vi "Draw Realtime.vi"(4 "Queue Items":i32, 5 "ColorRamp in":refnum<vi>, 6 "3D":T2, 7 "Resolution":i32=444, 8 "error in (no error)":errorcluster, 9 "Litho Point Old":T3, 10 "Litho Point":T3, 11 "Image in":T1(plugin-control)) -> (0 "error out":errorcluster, 3 "Image out":T1)   [LabVIEW 2016]
doc: "This VI draws on the realtime 2D and 3D images."
uses:
  <vilib>/vision/Image Controls.llb/IMAQ Image.ctl
  <vilib>/picture/3D Picture Control/Helpers/Apply Texture (no reference).vi
  <vilib>/picture/3D Picture Control/NI_3D Picture Control.lvlib
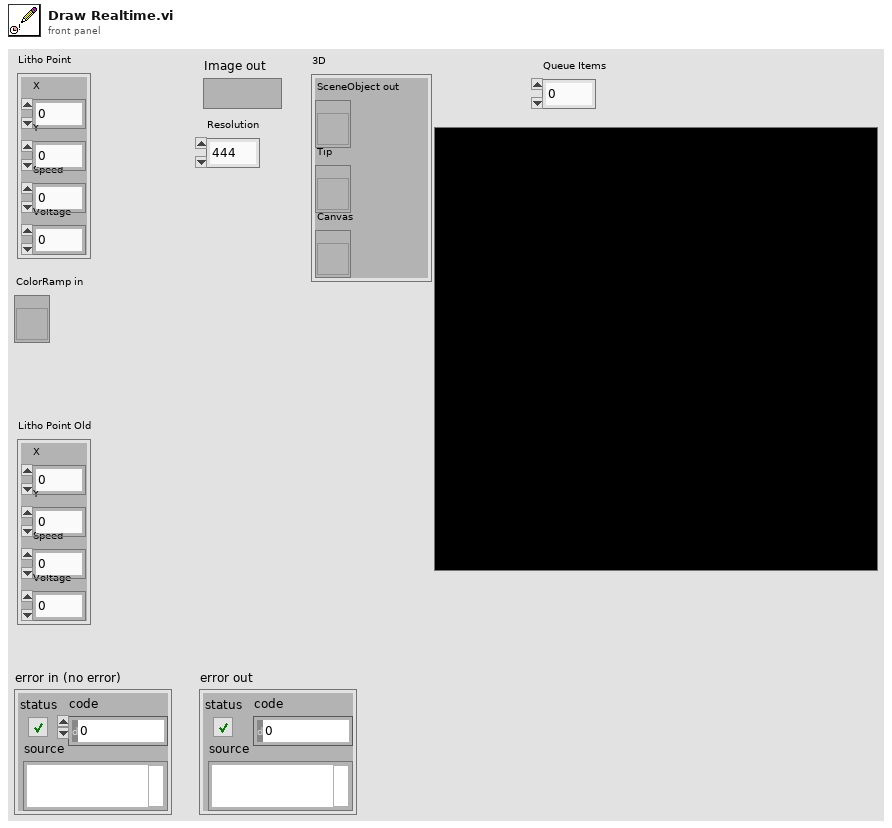
[diagram p1: front panel]
types:
  T1 = typedef "IMAQ Image.ctl" = refnum<image>
  T2 = cluster{"SceneObject out":refnum<vi>, "Tip":refnum<vi>, "Canvas":refnum<vi>}
  T3 = cluster{"X":dbl, "Y":dbl, "Speed":dbl, "Voltage":dbl}
  T4 = typedef "imagedata.ctl" = cluster{"image type":i32, "image depth":i32, "image":u8[], "mask":u8[], "colors":u32[], "Rectangle":cluster{"left":i16, "top":i16, "right":i16, "bottom":i16}}
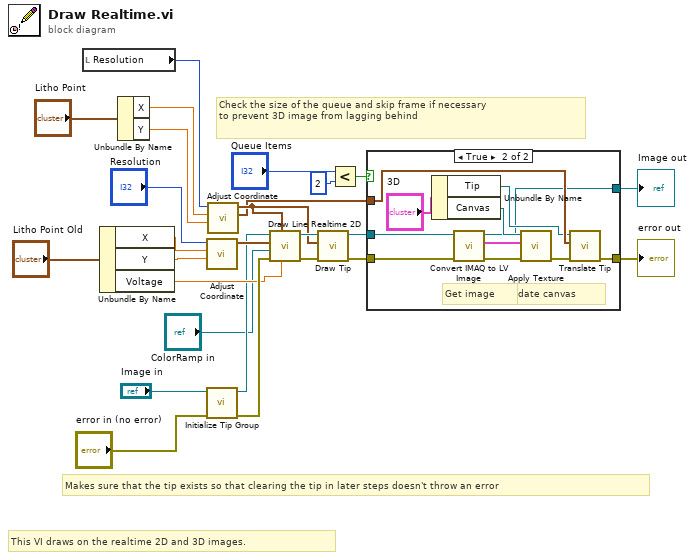
[diagram p0: block diagram]
diagram:
  # "This VI draws on the realtime 2D and 3D images."
  # "Makes sure that the tip exists so that clearing the tip in later steps doesn't throw an error"
  # "Check the size of the queue and skip frame if necessary\nto prevent 3D image from lagging behind"
  n1 = local read "Resolution"() -> (w3:i32)
  n2 = Unbundle By Name("Litho Point Old") -> ("X"=w24:dbl, "Y"=w25:dbl, "Voltage"=w12:dbl)
  n3 = Unbundle By Name("Litho Point") -> ("X"=w10:dbl, "Y"=w9:dbl)
  n4 = call "Adjust Coordinate.vi"("Y"=w25, "X"=w24, "Resolution"="Resolution") -> ("Adjusted Coordinate"=w23:cluster{dbl, dbl})  [unwired: 7 in, 1 out]
  n5 = call "Initialize Tip Group.vi"("error in (no error)"="error in (no error)", "Refnum in"="Image in") -> ("error out"=w19:errorcluster, "Refnum out"=w5:T1)  [unwired: 8 in]
  n6 = call "Adjust Coordinate.vi"("Y"=w9, "X"=w10, "Resolution"=w3) -> ("Offset Only"=w6:cluster{dbl, dbl}, "Adjusted Coordinate"=w7:cluster{dbl, dbl})  [unwired: 7 in]
  n7 = call "Draw Line Realtime 2D.vi"("Voltage"=w12, "Litho Point"=w7, "error in (no error)"=w19, "ColorRamp in"="ColorRamp in", "Litho Point Old"=w23, "Refnum in"=w5) -> ("error out"=w21:errorcluster, "Refnum out"=w22:T1)  [unwired: 4 in]
  n8 = call "Draw Tip.vi"("error in (no error)"=w21, "Adjusted Coordinate"=w7, "Refnum in"=w22) -> ("error out"=w17:errorcluster, "Refnum out"=w2:T1)  [unwired: 7 in]
  n9 = Less?(x="Queue Items", y=2) -> (x < y?=w13:bool)
  n10 = case shown="True" w13 {
    tunnel: w17 -> [w28 w38]
    tunnel: w6 -> [_ w35]
    tunnel: [w28 w34] -> w14
    tunnel: w2 -> [w27 w30]
    tunnel: [w27 w29] -> w1
    frame False {
    }
    frame True {
      # "Get image"
      # "Update canvas"
      n11 = Unbundle By Name("3D") -> ("Tip"=w31:refnum<vi>, "Canvas"=w32:refnum<vi>)
      n12 = call "Convert IMAQ to LV Image.vi"("error in (no error)"=w38, "IMAQImage In (RGB 32)"=w30) -> ("error out"=w37:errorcluster, "Output Image"=w39:T4, "IMAQImage Out"=w29:T1)  [unwired: 7 in]
      n13 = call-poly <vilib>:"Apply Texture.vi"("error in (no error)"=w37, "Image Data"=w39, "Scene Object In"=w32) -> ("error out"=w36:errorcluster)  [unwired: 7 in, 1 out]
      n14 = call "Translate Tip.vi"("error in (no error)"=w36, "Coordinate"=w35, "SceneObject in"=w31) -> ("error out"=w34:errorcluster)  [unwired: 8 in]
    }
  }
  "Image out" <- w1
  "error out" <- w14
